vi "Configure Scale Band Com.vi"(0 "VISA resource name":refnum<visa-resource-name>, 1 "Lower Position (0)":i32, 2 "Upper Position (1)":i32=1, 5 "Channel (001)":string="001", 7 "Area (0 : Off)":i32(ring) items=["Off", "In", "Out"], 9 "Color":cluster{"R":i32, "G":i32, "B":i32} {"B" min=0 max=255 step=1; "G" min=0 max=255 step=1; "R" min=0 max=255 step=1}, 11 "error in (no error)":errorcluster) -> (4 "VISA resource name out":refnum<visa-resource-name>, 6 "Channel":string, 15 "error out":errorcluster)   [LabVIEW 2020, in "Yokogawa GX Series.lvlib"]
doc: "Sets the green band of com channel."
uses:
  <instrlib>/Yokogawa GX Series/Yokogawa GX Series.lvlib
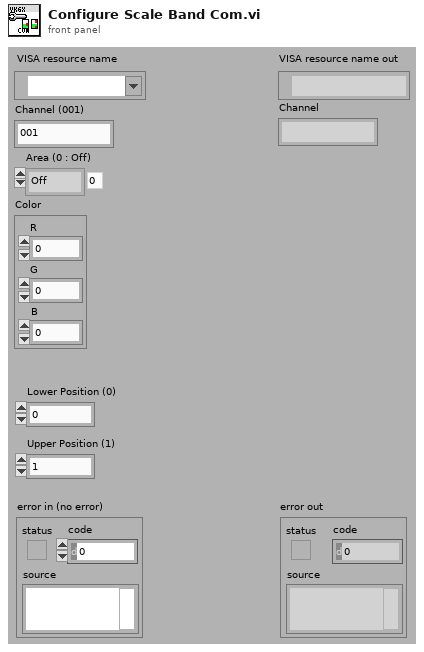
[diagram p1: front panel]
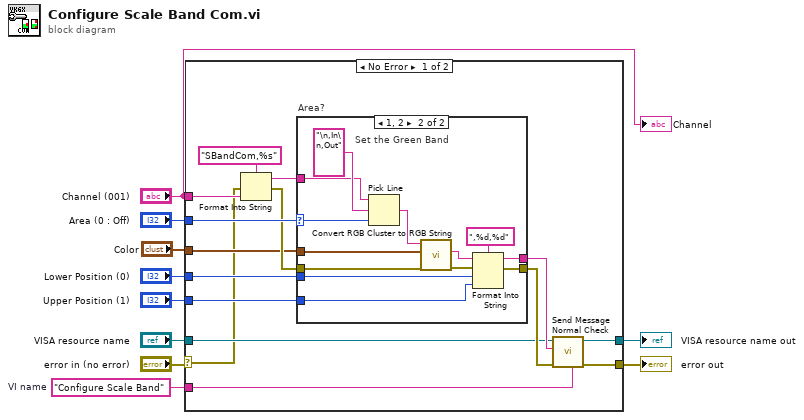
[diagram p0: block diagram]
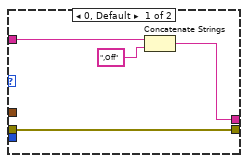
[diagram p2: hidden frame]
diagram:
  w2 = "Configure Scale Band"  # VI name
  n1 = case shown="No Error" "error in (no error)" {
    selector: "error in (no error)" -> [w11 w43]
    tunnel: "Area (0 : Off)" -> [w24 _]
    tunnel: "Lower Position (0)" -> [w21 _]
    tunnel: "Upper Position (1)" -> [w20 _]
    tunnel: "VISA resource name" -> [w17 w44]
    tunnel: [w16 w44] -> w6
    tunnel: [w15 w43] -> w5
    tunnel: "Color" -> [w14 _]
    tunnel: "Channel (001)" -> [w13 _]
    tunnel: w2 -> [w12 _]
    frame No Error {
      n2 = Format Into String(format string="SBandCom,%s", error in=w11, w13) -> (resulting string=w19:string, error out=w23:errorcluster)  [unwired: 1 in]
      n3 = case "Area?" shown="1, 2" w24 {
        selector: w24 -> [_ w36]
        tunnel: w23 -> [w29 w33]
        tunnel: [w29 w42] -> w22
        tunnel: w21 -> [_ w39]
        tunnel: w20 -> [_ w38]
        tunnel: [w26 w41] -> w18
        tunnel: w19 -> [w27 w35]
        tunnel: w14 -> [_ w34]
        frame 0, Default {
          n4 = Concatenate Strings(w27, ",Off") -> (w26:string)
        }
        frame 1, 2 {
          # "Set the Green Band"
          n5 = Pick Line(string ("")=w35, multi-line string="\n,In\n,Out" ("形式文字列"), line index=w36) -> (output string=w31:string)
          n6 = call <instrlib>:"Convert RGB Cluster to RGB String.vi"("error in (no error)"=w33, "RGB"=w34, "Initial String"=w31) -> ("error out"=w32:errorcluster, "RGB String"=w30:string)  [unwired: 7 in]
          n7 = Format Into String(format string=",%d,%d" ("形式文字列"), initial string=w30, error in=w32, w39, w38) -> (resulting string=w41:string, error out=w42:errorcluster)
        }
      }
      n8 = call <instrlib>:"Send Message Normal Check.vi"("Source (\"\")"=w12, "error in (no error)"=w22, "Send Message (\"\")"=w18, "VISA resource name"=w17) -> ("error out"=w15:errorcluster, "VISA resource name out"=w16:refnum<visa-resource-name>)  [unwired: 2 in, 4 out]
    }
    frame Error {
    }
  }
  "error out" <- w5
  "VISA resource name out" <- w6
  "Channel" <- "Channel (001)"
